vi "Phasor Check Type of Phasor Calculation.vi"(9 "# Gates":dbl, 10 "Gate Step":dbl[unit], 11 "Phasor Calculation in":T1) -> (1 "Changed?":bool, 3 "Phasor Calculation out":T1)   [LabVIEW 2021, in "Phasor.lvlib"]
uses:
  Phasor.lvlib
  Phasor Calculation Type.ctl
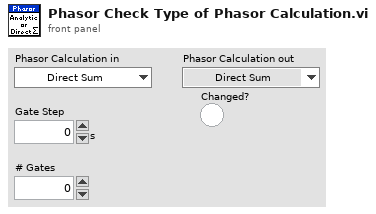
[diagram p1: front panel]
types:
  T1 = typedef "Phasor.lvlib/Phasor Calculation Type.ctl" = enum16{"Direct Sum", "Analytical Formula"}
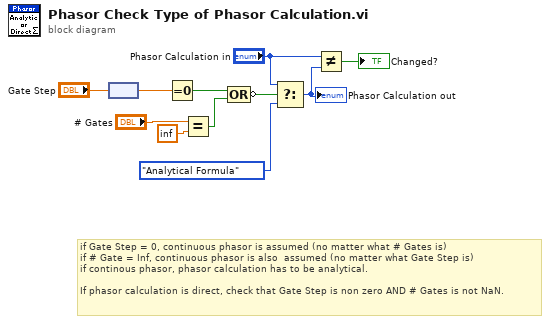
[diagram p0: block diagram]
diagram:
  # "if Gate Step = 0, continuous phasor is assumed (no matter what # Gates is)\nif # Gate = Inf, continuous phasor is also  assumed (no matter what Gate Step is)\nif continous phasor, phasor calculation has to be analytical.\n\nIf phasor calculation is direct, check that Gate Step is non zero AND # Gates is not NaN."
  n1 = node("Gate Step") -> (w2:dbl)
  n2 = Equal To 0?(x=w2) -> (x = 0?=w4:bool)
  n3 = Equal?(x="# Gates", y=inf) -> (x = y?=w5:bool)
  n4 = Compound Arithmetic op=OR(w4, w5) -> (invert w6:bool)
  n5 = Select(t="Phasor Calculation in", s=w6, f=Phasor_Calculation_Type."Analytical Formula") -> (s? t:f=w11:T1)
  "Phasor Calculation out" <- w11
  n6 = Not Equal?(x="Phasor Calculation in", y=w11) -> (x != y?=→"Changed?":bool)
